vi "ClusterwitharrayCDB.vi"(1 "Cluster In":cluster{"Array In":cdb[], "Numeric Input":cdb} {"Numeric Input" format="%.2f"; "Array In" format="%.2f"}, 2 "Base":cdb format="%.2f") -> (0 "Cluster Out":cluster{"Array Out":cdb[], "Numeric Output":cdb} {"Numeric Output" format="%.2f"; "Array Out" format="%.2f"})   [LabVIEW 2013]
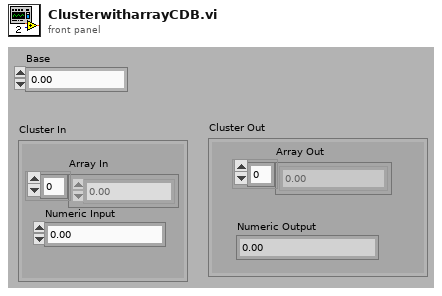
[diagram p1: front panel]
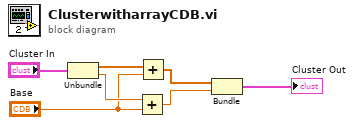
[diagram p0: block diagram]
diagram:
  n1 = Unbundle("Cluster In") -> ("Array In"=w6:cdb[], "Numeric Input"=w5:cdb)
  n2 = Add(x=w5, y="Base") -> (x+y=w1:cdb)
  n3 = Add(x=w6, y="Base") -> (x+y=w2:cdb[])
  n4 = Bundle(w2, w1) -> (→"Cluster Out":cluster{cdb[], cdb})  [unwired: 1 out]
